vi "Primary Flow.vi"(0 "Primary Delta T":dbl, 1 "Specific Heat Capacity of FLiBe":dbl, 2 "MHX Number of Tubes":dbl, 3 "Pipe Diameter":dbl, 4 "Pipe X-SectionArea":dbl, 5 "MHX Length":dbl, 6 "MHX Tube Diameter":dbl, 8 "Primary Average Temperature":dbl, 9 "Pri Hot Temp":dbl, 10 "Reactor Power":dbl, 11 "Pri Cold Temp":dbl, 12 "Time Interval (s)":dbl, 13 "Pri Mass Flow":dbl, 14 "MHX Heat Transfer":dbl) -> (16 "Pri Hot Temperature (K)":dbl, 18 "Thermal Driving Pressure (Pa)":dbl, 20 "Elbow Loss":dbl, 21 "Pri Cold Temperature (K)":dbl, 22 "Pressure Balance (Pa)":dbl, 23 "Pri Mass Flow (kg/s)":dbl, 24 "Pipe Loss":dbl, 25 "MHX Loss":dbl, 26 "RX Loss":dbl, 27 "HUR (C/min)":dbl)   [LabVIEW 2019]
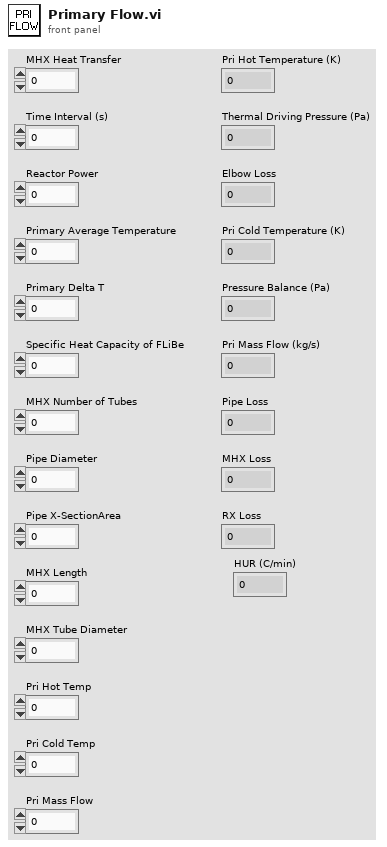
[diagram p1: front panel]
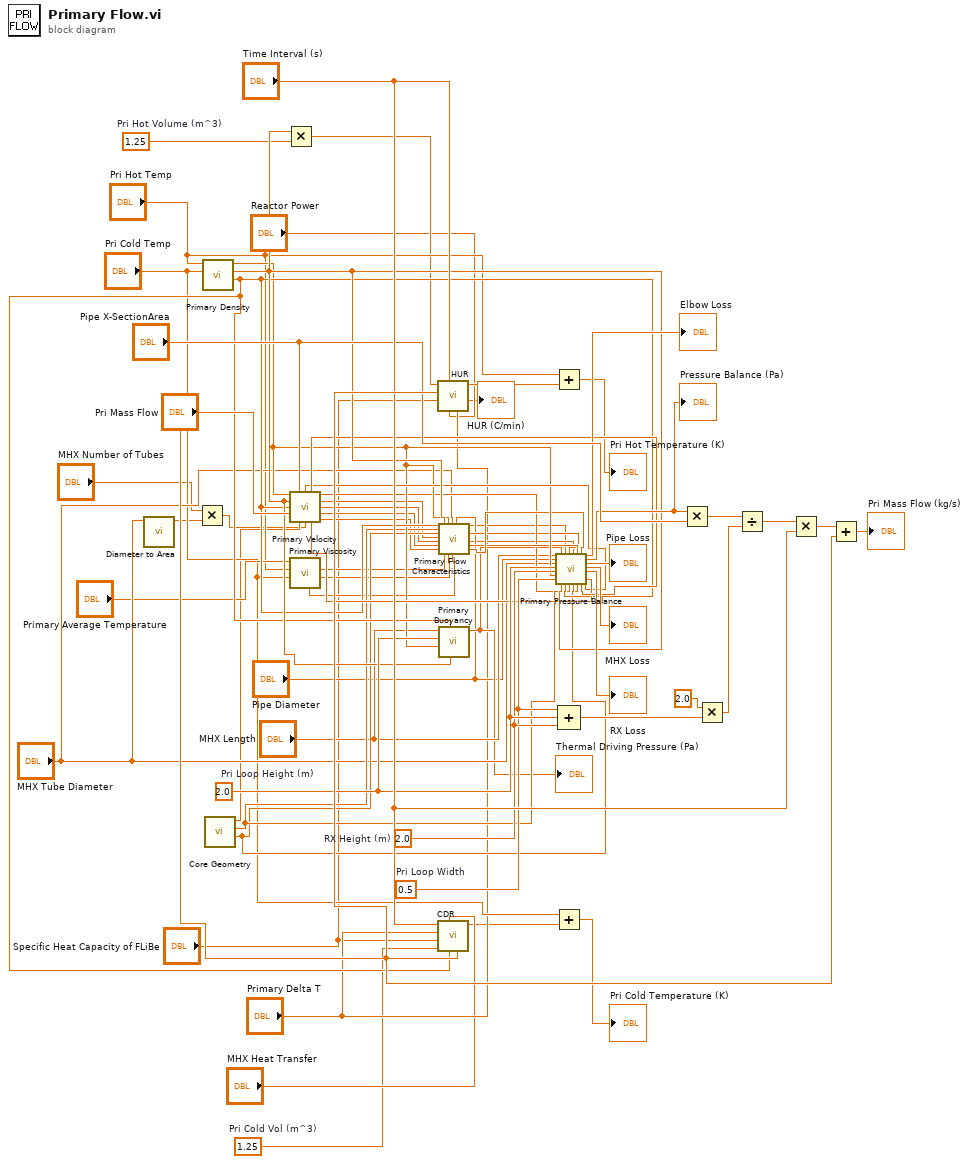
[diagram p0: block diagram]
diagram:
  w53 = 2.0  # RX Height (m)
  w52 = 0.5  # Pri Loop Width
  w54 = 2.0  # Pri Loop Height (m)
  w10 = 1.25  # Pri Hot Volume (m^3)
  w2 = 1.25  # Pri Cold Vol (m^3)
  n1 = call "Diameter to Area.vi"("Diameter (m)"="MHX Tube Diameter") -> ("Area (m^2)"=w14:dbl)  [unwired: 10 in]
  n2 = Multiply(x="MHX Number of Tubes", y=w14) -> (x*y=w15:dbl)
  n3 = call "Primary Density.vi"("Pri Cold Temp"="Pri Cold Temp", "Pri Hot Temp"="Pri Hot Temp") -> ("Primary Cold Density (kg/m^3)"=w41:dbl, "Primary Hot Density (kg/m^3)"=w44:dbl, "Primary Average Density (kg/m^3)"=w39:dbl)  [unwired: 7 in]
  n4 = call "Core Geometry.vi"() -> ("Downcomer Gap (m)"=w36:dbl, "Core Channel Equivalent Diameter (m)"=w38:dbl, "RX X-Section (m^2)"=w16:dbl)  [unwired: 9 in]
  n5 = Multiply(x=w44, y=w10) -> (x*y=w9:dbl)
  n6 = call "Primary Velocity.vi"("Primary Average Density"=w39, "Pipe X-SectionArea"="Pipe X-SectionArea", "Primary Hot Density"=w44, "Primary Cold Density"=w41, "Pri Mass Flow"="Pri Mass Flow", "RX X-Section"=w16, "Numeric"=w15) -> ("Cold Leg Velocity (m/s)"=w40:dbl, "Hot Leg Velocity (m/s)"=w43:dbl, "MHX Velocity (m/s)"=w34:dbl, "Velocity (m/s) 2"=w19:dbl, "Velocity (m/s) 4"=w17:dbl, "Velocity (m/s) 3"=w18:dbl, "RX Velocity (m/s)"=w42:dbl, "Velocity (m/s)"=w20:dbl)  [unwired: 1 in]
  n7 = call "Primary Viscosity.vi"("Pri Cold Temp"="Pri Cold Temp", "Pri Hot Temp"="Pri Hot Temp", "Primary Average Temperature"="Primary Average Temperature") -> ("FLiBe Viscosity (Pa-s) 2"=w25:dbl, "FLiBe Viscosity (Pa-s) 3"=w24:dbl, "FLiBe Viscosity (Pa-s)"=w26:dbl)  [unwired: 3 in, 3 out]
  n8 = call "HUR.vi"("Delta T (K)"="Primary Delta T", "Heating Power (W)"="Reactor Power", "Time"="Time Interval (s)", "Cp (J/kgK)"="Specific Heat Capacity of FLiBe", "Mass Flow (kg/s)"="Pri Mass Flow", "Hot Mass (kg)"=w9) -> ("HUR (C/min)"=→"HUR (C/min)":dbl, "HUR (K)"=w11:dbl)  [unwired: 3 in, 1 out]
  n9 = call "CDR.vi"("Mass Flow (kg/s)"="Pri Mass Flow", "Density (kg/m^3)"=w41, "HX Power (W)"="MHX Heat Transfer", "Cold Vol (m^3)"=w2, "Cp (J/kgK)"="Specific Heat Capacity of FLiBe", "Delta T (K)"="Primary Delta T", "Time (s)"="Time Interval (s)") -> ("Cooldown (K)"=w3:dbl)  [unwired: 4 in]
  n10 = call "Primary Flow Characteristics.vi"("Primary Cold Density"=w41, "Core Channel Equivalent Diameter"=w38, "Downcomer Gap"=w36, "Velocity (m/s) in"=w19, "Velocity (m/s) 4"=w17, "Velocity (m/s) 3"=w18, "Velocity"=w20, "Primary Hot Density"=w44, "FLiBe Viscosity (Pa-s) 3"=w24, "Primary Average Density"=w39, "FLiBe Viscosity (Pa-s) in"=w25, "MHX Tube Diameter"="MHX Tube Diameter", "FLiBe Viscosity"=w26, "Pipe Diameter"="Pipe Diameter") -> ("AC Friction Factor"=w27:dbl, "CD Friction Factor"=w31:dbl, "DF Friction Factor"=w28:dbl, "FG Friction Factor"=w35:dbl, "GA Friction Factor"=w37:dbl)  [unwired: 4 in, 5 out]
  n11 = call "Primary Buoyancy.vi"("Primary Hot Density"=w44, "Primary Cold Density"=w41, "Primary Average Density"=w39, "Pri Loop Height"=w54, "MHX Length"="MHX Length") -> ("Thermal Driving Pressure"=w30:dbl)  [unwired: 6 in]
  "Thermal Driving Pressure (Pa)" <- w30
  n12 = Add(x="Pri Hot Temp", y=w11) -> (x+y=→"Pri Hot Temperature (K)":dbl)
  n13 = Add(x="Pri Cold Temp", y=w3) -> (x+y=→"Pri Cold Temperature (K)":dbl)
  n14 = call "Primary Pressure Balance.vi"("MHX Length"="MHX Length", "Pipe Diameter"="Pipe Diameter", "MHX Tube Diameter"="MHX Tube Diameter", "Pri Loop Height"=w54, "RX Height"=w53, "Primary Average Density"=w39, "Pri Loop Width"=w52, "Thermal Driving Pressure"=w30, "Primary Hot Density"=w44, "AC Friction Factor"=w27, "Primary Cold Density"=w41, "CD Friction Factor"=w31, "Core Channel Equivalent Diameter"=w38, "DF Friction Factor"=w28, "Downcomer Gap"=w36, "FG Friction Factor"=w35, "MHX Velocity"=w34, "GA Friction Factor"=w37, "Hot Leg Velocity"=w43, "RX Velocity"=w42, "Cold Leg Velocity"=w40) -> ("Elbow Loss"=→"Elbow Loss":dbl, "Pressure Balance (Pa)"=w49:dbl, "Pipe Loss"=→"Pipe Loss":dbl, "MHX Loss"=→"MHX Loss":dbl, "RX Loss"=→"RX Loss":dbl)  [unwired: 2 in]
  "Pressure Balance (Pa)" <- w49
  n15 = Compound Arithmetic op=unknown(w52, w54, w53) -> (w56:dbl)
  n16 = Multiply(x=w49, y="Pipe X-SectionArea") -> (x*y=w51:dbl)
  n17 = Multiply(x=2.0, y=w56) -> (x*y=w55:dbl)
  n18 = Divide(x=w51, y=w55) -> (x/y=w58:dbl)
  n19 = Multiply(x=w58, y="Time Interval (s)") -> (x*y=w61:dbl)
  n20 = Add(x=w61, y="Pri Mass Flow") -> (x+y=→"Pri Mass Flow (kg/s)":dbl)
